vi "打印前面板R092C.vi"(0 "二维图片":picture) -> ()   [LabVIEW 2020]
panel:
  out "二维图片 2":picture
  # "P\n电动转向管柱\n带中间轴总成\n5045220000\n\nR092C-D622A-V012S"
  # "CHINA"
  # "P\n电动转向管柱\n带中间轴总成\n5045220000\n\nR092C-D622A-V012S"
  # "CHINA"
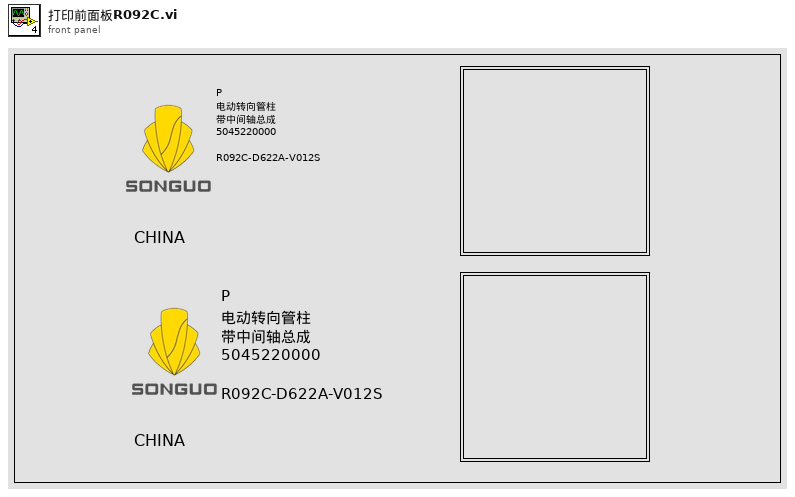
[diagram p1: front panel]
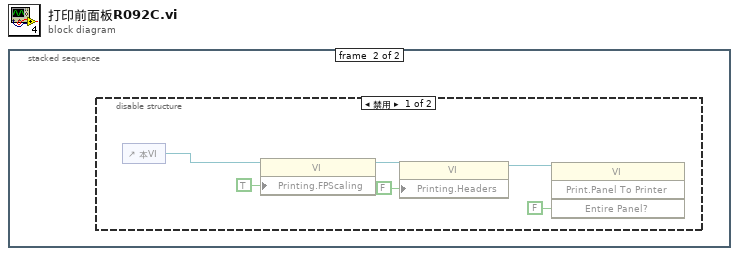
[diagram p0: block diagram]
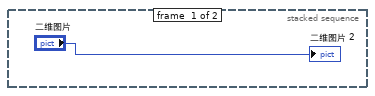
[diagram p2: hidden frame]
diagram:
  n1 = stacked-sequence {
    frame #0 {
      "二维图片 2" <- "二维图片"
    }
    frame #1 {
      n2 = disable-structure shown="禁用" {
        frame Disabled {
          n3 = control-ref of="本VI"() -> (w7:refnum<vi>)
          n4 = property class="VI"(reference=w7, "Printing.FPScaling"=TRUE ("打印:前面板缩放？")) -> (reference out=w5:refnum<vi>)  [unwired: 1 in, 1 out]
          n5 = property class="VI"(reference=w5, "Printing.Headers"=FALSE ("打印:页眉？")) -> (reference out=w3:refnum<vi>)  [unwired: 1 in, 1 out]
          n6 = invoke class="VI" method="Print.Panel To Printer"(reference=w3, "Entire Panel?"=FALSE ("整个前面板？")) -> ()  [unwired: 2 in, 4 out]
        }
        frame Enabled {
        }
      }
    }
  }
